vi "UHR-Fleezers Control (host) - 10.7.vi"() -> ()   [LabVIEW 2011] (continued)
        n1255 = Decrement(x="Scan steps (MCL)") -> (x-1=w1891:u64)
        n1256 = Divide(x="Scan Range (V)\n(of steps)", y=w1891) -> (x/y=w1890:dbl)
        "Desired Scan Incr (V)" <- w1890
        n1257 = local read "APD Integration Time (s)"() -> (w1883:dbl)
        n1258 = Multiply(x=w1890, y=w1870) -> (x*y=w1899:dbl)
        n1259 = Divide(x=w1899, y=10.0) -> (x/y=w1889:dbl)
        "Desired incr (int)" <- w1889
        n1260 = local read "Update Count (MCL)"() -> (w1895:u32)
        n1261 = Round Toward -Infinity(1:w1889) -> (0:w1898:dbl)
        n1262 = To Word Integer(number=w1898) -> (16bit integer=w1873:i16)
        "Actual Incr. int (MCL)" <- w1873
        n1263 = Multiply(x=w1883, y=40000000.0) -> (x*y=w1896:dbl)
        n1264 = Divide(x=w1896, y=w1895) -> (x/y=w1894:dbl)
        n1265 = Multiply(x=i16 10, y=w1873) -> (x*y=w1871:i16)
        n1266 = Multiply(x="N APD Samp/step", y=w1894) -> (x*y=w1893:dbl)
        "Cycles/step (MCL)" <- w1893
        n1267 = Divide(x=w1871, y=w1870) -> (x/y=→"Actual MCL Inc (V)":dbl)
        n1268 = Multiply(x="N APD Samp/step", y="Scan steps (MCL)") -> (x*y=w1885:dbl)
        n1269 = local read "APD Samples/FIFO Acq."() -> (w1882:dbl)
        n1270 = Multiply(x=w1885, y=u64 2) -> (x*y=w1884:dbl)
        "Data points/scan (f+b)" <- w1884
        n1271 = Multiply(x=w1884, y=w1875) -> (x*y=w1902:dbl)
        "Data points/scans (MCL)" <- w1902
        n1272 = Multiply(x=w1883, y=w1884) -> (x*y=w1876:dbl)
        "Time/f+b scan (s) (MCL)" <- w1876
        n1273 = Divide(x=w1902, y=w1882) -> (x/y=→"N sets should be saved (MCL)":dbl)
        n1274 = Multiply(x=w1876, y=w1875) -> (x*y=→"Total Time (s)":dbl)
        n1275 = Not(x="Fast Scan Dir") -> (.not. x?=w1880:bool)
        n1276 = xnode "Read/Write Control"("FPGA VI Reference In"=w1906, "error in"=w1905, "Scan steps (MCL)"="Scan steps (MCL)", "Number of scans (MCL)"=w1875, "Cycles per step (MCL)"=w1893, "Scan freq.  increment (MCL)"=w1873, "1D or 2D Scan?"="2D or 1D Scan", "MCL Scan Axis"=w1880, "Cont. Scan (MCL)"="Continuous MCL Scanning") -> ("error out"=w1904:errorcluster)  [unwired: 1 out]
      }
      event "Read Cal": Value Change {
        w1908 = 1000.0 ("y")
        n1277 = event-data() -> ()  [unwired: 7 out]
        n1278 = local read "Save file name"() -> (w1933:path)
        n1279 = local write "Read Cal"(FALSE ("Read Cal")) -> ()
        n1280 = Strip Path(path=w1933) -> (stripped path=w1932:path)  [unwired: 1 out]
        n1281 = Path To String(path=w1932) -> (string=w1931:string)
        n1282 = Concatenate Strings(w1931, "\\current.cal" ("string")) -> (w1929:string)
        n1283 = String To Path(string=w1929) -> (path=w1928:path)
        n1284 = Open/Create/Replace File(file path (use dialog)=w1928, operation (0:open)=T25."open", access (0:read/write)=enum16{"read/write", "read-only", "write-only"}."read-only") -> (refnum out=w1936:refnum<file>, error out=w1922:errorcluster)  [unwired: 1 in, 3 out]
        n1285 = Deny Access(4:w1922, 7:w1936) -> (0:w1921:errorcluster, 3:w1927:refnum<file>)  [unwired: 1 out]
        n1286 = Read from Binary File(5:0.0, 8:w1921, 9:T24."big-endian, network order" ("byte order (0:big-endian, network order)"), 10:-1 ("count (1)"), 11:w1927) -> (0:w1920:errorcluster, 2:w1918:dbl[], 3:w1923:refnum<file>)  [unwired: 2 out]
        n1287 = Array To Cluster(array=w1918) -> (cluster=w1917:T27)
        n1288 = Unbundle(w1917) -> ("[0]"=w1916:dbl, "[1]"=w1915:dbl, "[2]"=w1914:dbl, "[3]"=w1913:dbl, "[4]"=w1912:dbl, "[5]"=w1911:dbl)
        n1289 = Close File(refnum=w1923, error in=w1920) -> (error out=→"Read cal error":errorcluster)  [unwired: 1 out]
        n1290 = Multiply(x=w1911, y=w1908) -> (x*y=w1909:dbl)
        n1291 = local write "T2 kappa_x (pN/nm)"(w1913) -> ()
        n1292 = local write "T1 kappa_x (pN/nm)"(w1914) -> ()
        n1293 = local write "T1 alpha_x (nm/V)"(w1916) -> ()
        n1294 = local write "T2 alpha_x (nm/V)"(w1915) -> ()
        n1295 = Multiply(x=w1912, y=w1908) -> (x*y=w1910:dbl)
        n1296 = local write "T1 offset_x (mV)"(w1910) -> ()
        n1297 = local write "T2 offset_x (mV)"(w1909) -> ()
      }
      event "Abort MCL Scan": Value Change {
        n1298 = event-data() -> ()  [unwired: 7 out]
        n1299 = local write "MCL Scanning"(FALSE ("MCL Scanning")) -> ()
        n1300 = xnode "Read/Write Control"("FPGA VI Reference In"=w1941, "error in"=w1940, "Abort scan (MCL)"="Abort MCL Scan") -> ("error out"=w1939:errorcluster)  [unwired: 1 out]
      }
      event "Update Count (MCL)": Value Change {
        n1301 = event-data() -> ()  [unwired: 7 out]
        n1302 = xnode "Read/Write Control"("FPGA VI Reference In"=w1945, "error in"=w1944, "MCL count"="Update Count (MCL)") -> ("error out"=w1943:errorcluster)  [unwired: 1 out]
      }
      event "Phase adjust (MCL)", "+ phase (MCL)", "- phase (MCL)": Value Change {
        n1303 = event-data() -> ()  [unwired: 7 out]
        n1304 = Negate(x="Phase adjust (MCL)") -> (-x=w1954:i16)
        n1305 = Select(t=w1954, s="- phase (MCL)", f="Phase adjust (MCL)") -> (s? t:f=w1952:i16)
        n1306 = Or(x="- phase (MCL)", y="+ phase (MCL)") -> (x .or. y?=w1947:bool)
        n1307 = xnode "Read/Write Control"("FPGA VI Reference In"=w1956, "error in"=w1955, "Phase count adjustment (MCL)"=w1952) -> ("FPGA VI Reference Out"=w1948:T19, "error out"=w1949:errorcluster)
        n1308 = xnode "Read/Write Control"("FPGA VI Reference In"=w1948, "error in"=w1949, "+ phase (MCL)"=w1947) -> ("error out"=w1946:errorcluster)  [unwired: 1 out]
      }
      event "Abort AOD Scan": Value Change {
        n1309 = event-data() -> ()  [unwired: 7 out]
        n1310 = xnode "Read/Write Control"("FPGA VI Reference In"=w1960, "error in"=w1959, "Abort scan"="Abort AOD Scan") -> ("error out"=w1958:errorcluster)  [unwired: 1 out]
      }
      event "Continuous AOD Scanning": Value Change {
        n1311 = event-data() -> ()  [unwired: 7 out]
        n1312 = xnode "Read/Write Control"("FPGA VI Reference In"=w1964, "error in"=w1963, "Cont. Scan"="Continuous AOD Scanning") -> ("error out"=w1962:errorcluster)  [unwired: 1 out]
      }
      event "Index": Value Change {
        n1313 = event-data() -> ()  [unwired: 7 out]
        n1314 = call "Create new save file.vi"("Insert"="", "Ext"=".dat" ("string"), "Index In"="Index") -> ("Path Out"=→"Save file name":path, "Index Out"=w1965:dbl)
        "Save index" <- w1965
        n1315 = local write "Index"(w1965) -> ()
      }
      event "AO1", "AO2": Value Change {
        w1980 = 10.0 ("y")
        w1979 = 32767.0 ("y")
        n1316 = event-data() -> ()  [unwired: 7 out]
        n1317 = local read "AO2"() -> (w1978:dbl)
        n1318 = local read "AO1"() -> (w1975:dbl)
        n1319 = Multiply(x=w1975, y=w1979) -> (x*y=w1974:dbl)
        n1320 = Multiply(x=w1978, y=w1979) -> (x*y=w1977:dbl)
        n1321 = Divide(x=w1974, y=w1980) -> (x/y=w1973:dbl)
        n1322 = Divide(x=w1977, y=w1980) -> (x/y=w1976:dbl)
        n1323 = To Word Integer(number=w1973) -> (16bit integer=w1981:i16)
        n1324 = To Word Integer(number=w1976) -> (16bit integer=w1982:i16)
        n1325 = xnode "Read/Write Control"("FPGA VI Reference In"=w1972, "error in"=w1971, "AO1"=w1981, "AO2"=w1982) -> ("error out"=w1970:errorcluster)  [unwired: 1 out]
      }
      event "Inject Pump 1": Value Change {
        n1326 = event-data() -> ()  [unwired: 7 out]
        n1327 = local read "Use Harvard pumps\nfor beads (else Chemyx)"() -> (w1984:bool)
        n1328 = case shown="True" w1984 {
          tunnel: "Inject Pump 1" -> [w1988 w2026]
          tunnel: w1983 -> [_ w2027]
          frame False {
            n1329 = local read "Pump write delay (ms)"() -> (w1987:dbl)
            n1330 = local read "Chemyx Syringe Pump Serial Port"() -> (w1986:refnum<visa-resource-name>)
            n1331 = case shown="True" w1988 {
              tunnel: w1987 -> [w1994 w2008]
              tunnel: w1986 -> [w1991 w2007]
              frame False {
                n1332 = flat-sequence {
                  tunnel: w1991 -> [w1995]
                  tunnel: [w1995] -> w1992
                  tunnel: w1994 -> [_]
                  tunnel: [w1998] -> w1993
                  tunnel: w1992 -> [w1998]
                  tunnel: w1993 -> [w1999]
                  tunnel: [w1999] -> w1989
                  tunnel: [w2001] -> w1990
                  tunnel: w1989 -> [w2001]
                  tunnel: w1990 -> [w2003]
                  frame #0 {
                    n1333 = call "Write to pump.vi"("string"="enter pump1", "VISA resource name"=w1995) -> ()  [unwired: 1 out]
                  }
                  frame #1 {
                    n1334 = Wait (ms)(milliseconds to wait="Pump pause delay (ms)") -> ()  [unwired: 1 out]
                  }
                  frame #2 {
                    n1335 = call "Write to pump.vi"("string"="stop", "VISA resource name"=w1999) -> ()  [unwired: 1 out]
                  }
                  frame #3 {
                    n1336 = Wait (ms)(milliseconds to wait=u32 500) -> ()  [unwired: 1 out]
                  }
                  frame #4 {
                    n1337 = call "Write to pump.vi"("string"="stop", "VISA resource name"=w2003) -> ()  [unwired: 1 out]
                  }
                }
              }
              frame True {
                n1338 = flat-sequence {
                  tunnel: w2007 -> [w2017]
                  tunnel: w2008 -> [w2012]
                  tunnel: w2008 -> [w2019]
                  tunnel: w2007 -> [w2020]
                  tunnel: [w2020] -> w2005
                  tunnel: [w2022] -> w2006
                  tunnel: w2005 -> [w2022]
                  tunnel: w2006 -> [w2024]
                  frame #0 {
                    n1339 = local read "All Pump Parameters"() -> (w2011:T5)
                    n1340 = Unbundle By Name(w2011) -> ("Pump 1"=w2018:T28)
                    n1341 = call "Set pump parameters.vi"("Pump write delay (ms)"=w2012, "Volume (uL)"="Ch 1 Inject Volume (uL)", "Rate (uL/h)"="Ch 1 Inject Rate (ul/h)", "Units"=4.0, "Pump #"=1.0, "Pump Parameters In"=w2018, "VISA resource name"=w2017) -> ("Pump Parameters Out"=w2010:T28)  [unwired: 3 in]
                    n1342 = Bundle By Name(cluster=w2011, "Pump 1"=w2010) -> (w2009:T5)
                    n1343 = local write "All Pump Parameters"(w2009) -> ()
                  }
                  frame #1 {
                    n1344 = Wait (ms)(milliseconds to wait=w2019) -> ()  [unwired: 1 out]
                  }
                  frame #2 {
                    n1345 = call "Write to pump.vi"("string"="start", "VISA resource name"=w2020) -> ()  [unwired: 1 out]
                  }
                  frame #3 {
                    n1346 = Wait (ms)(milliseconds to wait=u32 500) -> ()  [unwired: 1 out]
                  }
                  frame #4 {
                    n1347 = call "Write to pump.vi"("string"="start", "VISA resource name"=w2024) -> ()  [unwired: 1 out]
                  }
                }
              }
            }
          }
          frame True {
            n1348 = case shown="False" w2026 {
              tunnel: w2027 -> [w2028 w2038]
              frame False {
                n1349 = flat-sequence {
                  tunnel: w2028 -> [w2030]
                  frame #0 {
                    n1350 = local write "Flushing P1"(FALSE ("Flushing P1")) -> ()
                    n1351 = Concatenate Strings("stop" ("string"), "\r") -> (w2032:string)
                    n1352 = VISA Write(VISA resource name=w2030, write buffer=w2032) -> ()  [unwired: 1 in, 3 out]
                  }
                  frame #1 {
                    n1353 = property on="Clear Volume P1" class="Bool (strict)"("Val(Sgnl)"=TRUE ("Value (Signaling)")) -> ()  [unwired: 2 in, 2 out]
                  }
                }
              }
              frame True {
                n1354 = local read "Normal Flow Rate (ul/h) P1"() -> (w2036:dbl)
                n1355 = Number To Decimal String(number=w2036) -> (decimal integer string=w2042:string)  [unwired: 1 in]
                n1356 = Concatenate Strings("irate  " ("string"), w2042, " u/h" ("string"), "\r") -> (w2040:string)
                n1357 = VISA Write(VISA resource name=w2038, write buffer=w2040) -> (VISA resource name out=w2037:refnum<visa-resource-name>)  [unwired: 1 in, 2 out]
                n1358 = Concatenate Strings("irun" ("string"), "\r") -> (w2044:string)
                n1359 = VISA Write(VISA resource name=w2037, write buffer=w2044) -> ()  [unwired: 1 in, 3 out]
              }
            }
          }
        }
      }
      event "Inject Pump 3": Value Change {
        n1360 = event-data() -> ()  [unwired: 7 out]
        n1361 = local read "Use Harvard pumps\nfor beads (else Chemyx)"() -> (w2047:bool)
        n1362 = case shown="True" w2047 {
          tunnel: "Inject Pump 3" -> [w2051 w2090]
          tunnel: w2046 -> [_ w2089]
          frame False {
            n1363 = local read "Pump write delay (ms)"() -> (w2050:dbl)
            n1364 = case shown="True" w2051 {
              tunnel: w2050 -> [w2057 w2071]
              tunnel: "Chemyx Syringe Pump Serial Port" -> [w2054 w2070]
              frame False {
                n1365 = flat-sequence {
                  tunnel: w2054 -> [w2058]
                  tunnel: [w2058] -> w2055
                  tunnel: w2057 -> [_]
                  tunnel: [w2061] -> w2056
                  tunnel: w2055 -> [w2061]
                  tunnel: w2056 -> [w2062]
                  tunnel: [w2062] -> w2052
                  tunnel: [w2064] -> w2053
                  tunnel: w2052 -> [w2064]
                  tunnel: w2053 -> [w2066]
                  frame #0 {
                    n1366 = call "Write to pump.vi"("string"="enter pump3", "VISA resource name"=w2058) -> ()  [unwired: 1 out]
                  }
                  frame #1 {
                    n1367 = local read "Pump pause delay (ms)"() -> (w2060:u32)
                    n1368 = Wait (ms)(milliseconds to wait=w2060) -> ()  [unwired: 1 out]
                  }
                  frame #2 {
                    n1369 = call "Write to pump.vi"("string"="stop", "VISA resource name"=w2062) -> ()  [unwired: 1 out]
                  }
                  frame #3 {
                    n1370 = Wait (ms)(milliseconds to wait=u32 0) -> ()  [unwired: 1 out]
                  }
                  frame #4 {
                    n1371 = call "Write to pump.vi"("string"="stop", "VISA resource name"=w2066) -> ()  [unwired: 1 out]
                  }
                }
              }
              frame True {
                n1372 = flat-sequence {
                  tunnel: w2070 -> [w2080]
                  tunnel: w2071 -> [w2075]
                  tunnel: w2071 -> [w2082]
                  tunnel: w2070 -> [w2083]
                  tunnel: [w2083] -> w2069
                  tunnel: [w2086] -> w2068
                  tunnel: w2069 -> [w2086]
                  tunnel: w2068 -> [w2087]
                  frame #0 {
                    n1373 = local read "All Pump Parameters"() -> (w2074:T5)
                    n1374 = Unbundle By Name(w2074) -> ("Pump 3"=w2081:T28)
                    n1375 = call "Set pump parameters.vi"("Pump write delay (ms)"=w2075, "Volume (uL)"="Ch 3 Inject Volume (uL)", "Rate (uL/h)"="Ch 3 Inject Rate (ul/h)", "Units"=4.0, "Pump #"=3.0, "Pump Parameters In"=w2081, "VISA resource name"=w2080) -> ("Pump Parameters Out"=w2073:T28)  [unwired: 3 in]
                    n1376 = Bundle By Name(cluster=w2074, "Pump 3"=w2073) -> (w2072:T5)
                    n1377 = local write "All Pump Parameters"(w2072) -> ()
                  }
                  frame #1 {
                    n1378 = Wait (ms)(milliseconds to wait=w2082) -> ()  [unwired: 1 out]
                  }
                  frame #2 {
                    n1379 = call "Write to pump.vi"("string"="start", "VISA resource name"=w2083) -> ()  [unwired: 1 out]
                  }
                  frame #3 {
                    n1380 = Wait (ms)(milliseconds to wait=u32 500) -> ()  [unwired: 1 out]
                  }
                  frame #4 {
                    n1381 = call "Write to pump.vi"("string"="start", "VISA resource name"=w2087) -> ()  [unwired: 1 out]
                  }
                }
              }
            }
          }
          frame True {
            n1382 = case shown="False" w2090 {
              tunnel: w2089 -> [w2091 w2098]
              frame False {
                n1383 = flat-sequence {
                  tunnel: w2091 -> [w2093]
                  frame #0 {
                    n1384 = local write "Flushing P3"(FALSE ("Flushing P3")) -> ()
                    n1385 = Concatenate Strings("stop" ("string"), "\r") -> (w2095:string)
                    n1386 = VISA Write(VISA resource name=w2093, write buffer=w2095) -> ()  [unwired: 1 in, 3 out]
                  }
                  frame #1 {
                    n1387 = property on="Clear Volume P3" class="Bool (strict)"("Val(Sgnl)"=TRUE ("Value (Signaling)")) -> ()  [unwired: 2 in, 2 out]
                  }
                }
              }
              frame True {
                n1388 = local read "Normal Flow Rate (ul/h) P3"() -> (w2099:dbl)
                n1389 = Number To Decimal String(number=w2099) -> (decimal integer string=w2105:string)  [unwired: 1 in]
                n1390 = Concatenate Strings("irate  " ("string"), w2105, " u/h" ("string"), "\r") -> (w2103:string)
                n1391 = VISA Write(VISA resource name=w2098, write buffer=w2103) -> (VISA resource name out=w2101:refnum<visa-resource-name>)  [unwired: 1 in, 2 out]
                n1392 = Concatenate Strings("irun" ("string"), "\r") -> (w2107:string)
                n1393 = VISA Write(VISA resource name=w2101, write buffer=w2107) -> ()  [unwired: 1 in, 3 out]
              }
            }
          }
        }
      }
      event "Inject Pump 2": Value Change {
        n1394 = event-data() -> ()  [unwired: 7 out]
        n1395 = local read "Pump write delay (ms)"() -> (w2111:dbl)
        n1396 = flat-sequence {
          tunnel: w2109 -> [w2124]
          tunnel: w2111 -> [w2120]
          tunnel: "Inject Pump 2" -> [_]
          tunnel: w2111 -> [w2126]
          tunnel: w2109 -> [w2127]
          frame #0 {
            n1397 = local read "All Pump Parameters"() -> (w2119:T5)
            n1398 = Multiply(x=60.0, y="Flush Center Ch Rate (ul/m)") -> (x*y=w2116:dbl)
            n1399 = Unbundle By Name(w2119) -> ("Pump 2"=w2125:T28)
            n1400 = call "Set pump parameters.vi"("Pump write delay (ms)"=w2120, "Volume (uL)"="Flush Center Ch Volume (uL)", "Rate (uL/h)"=w2116, "Units"=3.0, "Pump #"=2.0, "Pump Parameters In"=w2125, "VISA resource name"=w2124) -> ("Pump Parameters Out"=w2118:T28)  [unwired: 3 in]
            n1401 = Bundle By Name(cluster=w2119, "Pump 2"=w2118) -> (w2117:T5)
            n1402 = local write "All Pump Parameters"(w2117) -> ()
            n1403 = Add(x="Flush Center Ch Volume (uL)", y="Total Volume\nFlushed (uL)") -> (x+y=w2113:dbl)
            n1404 = local write "Total Volume\nFlushed (uL)"(w2113) -> ()
          }
          frame #1 {
            n1405 = Wait (ms)(milliseconds to wait=w2126) -> ()  [unwired: 1 out]
          }
          frame #2 {
            n1406 = call "Write to pump.vi"("string"="start", "VISA resource name"=w2127) -> ()  [unwired: 1 out]
          }
        }
        n1407 = local read "Chemyx Syringe Pump Serial Port"() -> (w2109:refnum<visa-resource-name>)
      }
      event "Sample Channel\nFlow": Value Change {
        n1408 = event-data() -> ()  [unwired: 7 out]
        n1409 = Select(t="irun" ("string"), s="Sample Channel\nFlow", f="stop" ("string")) -> (s? t:f=w2131:string)
        n1410 = Concatenate Strings(w2131, "\r") -> (w2134:string)
        n1411 = VISA Write(VISA resource name=w2129, write buffer=w2134) -> ()  [unwired: 1 in, 3 out]
      }
      event "Start Flow": Value Change {
        n1412 = event-data() -> ()  [unwired: 7 out]
        n1413 = local write "Sample Channel\nFlow"(TRUE ("Sample Channel\nFlow")) -> ()
        n1414 = local write "Start Flow"(FALSE ("Start Flow")) -> ()
        n1415 = Concatenate Strings("irun" ("string"), "\r") -> (w2140:string)
        n1416 = VISA Write(VISA resource name=w2136, write buffer=w2140) -> ()  [unwired: 1 in, 3 out]
      }
      event "Stop Flow": Value Change {
        w2142 = FALSE ("Stop Flow")
        n1417 = event-data() -> ()  [unwired: 7 out]
        n1418 = local write "Stop Flow"(w2142) -> ()
        n1419 = local write "Sample Channel\nFlow"(w2142) -> ()
        n1420 = Concatenate Strings("stop" ("string"), "\r") -> (w2145:string)
        n1421 = VISA Write(VISA resource name=w2143, write buffer=w2145) -> ()  [unwired: 1 in, 3 out]
      }
      event "Flow rate (uL/h)": Value Change {
        n1422 = event-data() -> ()  [unwired: 7 out]
        n1423 = Number To Decimal String(number="Flow rate (uL/h)") -> (decimal integer string=w2152:string)  [unwired: 1 in]
        n1424 = Concatenate Strings("irate  " ("string"), w2152, " u/h" ("string"), "\r") -> (w2151:string)
        n1425 = VISA Write(VISA resource name=w2148, write buffer=w2151) -> ()  [unwired: 1 in, 3 out]
      }
      event "Flush Sample": Value Change {
        n1426 = event-data() -> ()  [unwired: 7 out]
        n1427 = flat-sequence {
          tunnel: w2157 -> [w2185]
          tunnel: [w2165] -> w2156
          tunnel: [w2159] -> w2154
          tunnel: w2156 -> [w2189]
          tunnel: [w2189] -> w2155
          tunnel: w2154 -> [w2188]
          tunnel: w2155 -> [w2194]
          frame #0 {
            # "set paramaters (rate, volume) for flush, clear volume"
            n1428 = Number To Decimal String(number="Flush rate (uL/m)") -> (decimal integer string=w2181:string)  [unwired: 1 in]
            n1429 = Concatenate Strings("irate  " ("string"), w2181, " u/m" ("string"), "\r") -> (w2183:string)
            n1430 = VISA Write(VISA resource name=w2185, write buffer=w2183) -> (VISA resource name out=w2179:refnum<visa-resource-name>)  [unwired: 1 in, 2 out]
            n1431 = Reciprocal(x="Flush rate (uL/m)") -> (1/x=w2162:dbl)
            n1432 = Number To Decimal String(number="Volume (uL)") -> (decimal integer string=w2170:string)  [unwired: 1 in]
            n1433 = Multiply(x="Volume (uL)", y=w2162) -> (x*y=w2161:dbl)
            n1434 = Concatenate Strings("tvolume  " ("string"), w2170, " u" ("string"), "\r") -> (w2168:string)
            n1435 = Multiply(x=w2161, y=60000.0) -> (x*y=w2159:dbl)
            n1436 = VISA Write(VISA resource name=w2179, write buffer=w2168) -> (VISA resource name out=w2167:refnum<visa-resource-name>)  [unwired: 1 in, 2 out]
            n1437 = Concatenate Strings("cvolume" ("string"), "\r") -> (w2166:string)
            n1438 = VISA Write(VISA resource name=w2167, write buffer=w2166) -> (VISA resource name out=w2177:refnum<visa-resource-name>)  [unwired: 1 in, 2 out]
            n1439 = Concatenate Strings("irun" ("string"), "\r") -> (w2175:string)
            n1440 = VISA Write(VISA resource name=w2177, write buffer=w2175) -> (VISA resource name out=w2165:refnum<visa-resource-name>)  [unwired: 1 in, 2 out]
          }
          frame #1 {
            # "Have to wait until\nflow is done to reset\nrate"
            n1441 = Add(x=w2188, y=100.0) -> (x+y=w2187:dbl)
            n1442 = Wait (ms)(milliseconds to wait=w2187) -> ()  [unwired: 1 out]
          }
          frame #2 {
            # "reset flow rate to usual flow rate"
            n1443 = local read "Flow rate (uL/h)"() -> (w2200:dbl)
            n1444 = Number To Decimal String(number=w2200) -> (decimal integer string=w2198:string)  [unwired: 1 in]
            n1445 = Concatenate Strings("irate  " ("string"), w2198, " u/h" ("string"), "\r") -> (w2196:string)
            n1446 = VISA Write(VISA resource name=w2194, write buffer=w2196) -> (VISA resource name out=w2190:refnum<visa-resource-name>)  [unwired: 1 in, 2 out]
            n1447 = Concatenate Strings("cvolume" ("string"), "\r") -> (w2191:string)
            n1448 = VISA Write(VISA resource name=w2190, write buffer=w2191) -> ()  [unwired: 1 in, 3 out]
          }
        }
      }
      event "Flush Pump 3": Value Change {
        n1449 = event-data() -> ()  [unwired: 7 out]
        n1450 = flat-sequence {
          tunnel: w2201 -> [w2204]
          frame #0 {
            # "set paramaters (rate, volume) for flush, clear volume"
            n1451 = Number To Decimal String(number="Flush rate (uL/m) P3") -> (decimal integer string=w2226:string)  [unwired: 1 in]
            n1452 = local write "Inject Pump 3"(TRUE ("Inject Pump 3")) -> ()
            n1453 = Concatenate Strings("irate  " ("string"), w2226, " u/m" ("string"), "\r") -> (w2228:string)
            n1454 = VISA Write(VISA resource name=w2204, write buffer=w2228) -> (VISA resource name out=w2224:refnum<visa-resource-name>)  [unwired: 1 in, 2 out]
            n1455 = Reciprocal(x="Flush rate (uL/m) P3") -> (1/x=w2208:dbl)
            n1456 = Number To Decimal String(number="Volume (uL) P3") -> (decimal integer string=w2215:string)  [unwired: 1 in]
            n1457 = Multiply(x="Volume (uL) P3", y=w2208) -> (x*y=w2207:dbl)
            n1458 = Concatenate Strings("tvolume  " ("string"), w2215, " u" ("string"), "\r") -> (w2213:string)
            n1459 = Multiply(x=w2207, y=60.0) -> (x*y=→"HP3 Flush Time (s)":dbl)
            n1460 = VISA Write(VISA resource name=w2224, write buffer=w2213) -> (VISA resource name out=w2212:refnum<visa-resource-name>)  [unwired: 1 in, 2 out]
            n1461 = Concatenate Strings("cvolume" ("string"), "\r") -> (w2211:string)
            n1462 = VISA Write(VISA resource name=w2212, write buffer=w2211) -> (VISA resource name out=w2222:refnum<visa-resource-name>)  [unwired: 1 in, 2 out]
            n1463 = Concatenate Strings("irun" ("string"), "\r") -> (w2220:string)
            n1464 = VISA Write(VISA resource name=w2222, write buffer=w2220) -> ()  [unwired: 1 in, 3 out]
          }
          frame #1 {
            "Flushing P3" <- TRUE ("Flushing P3")
          }
        }
      }
      event "Flush Pump 1": Value Change {
        n1465 = event-data() -> ()  [unwired: 7 out]
        n1466 = flat-sequence {
          tunnel: [w2242] -> w2232
          tunnel: w2231 -> [w2235]
          tunnel: w2232 -> [_]
          frame #0 {
            # "set paramaters (rate, volume) for flush, clear volume"
            n1467 = local write "Inject Pump 1"(TRUE ("Inject Pump 1")) -> ()
            n1468 = Number To Decimal String(number="Flush rate (uL/m) P1") -> (decimal integer string=w2258:string)  [unwired: 1 in]
            n1469 = Concatenate Strings("irate  " ("string"), w2258, " u/m" ("string"), "\r") -> (w2260:string)
            n1470 = VISA Write(VISA resource name=w2235, write buffer=w2260) -> (VISA resource name out=w2256:refnum<visa-resource-name>)  [unwired: 1 in, 2 out]
            n1471 = Reciprocal(x="Flush rate (uL/m) P1") -> (1/x=w2239:dbl)
            n1472 = Number To Decimal String(number="Volume (uL) P1") -> (decimal integer string=w2247:string)  [unwired: 1 in]
            n1473 = Multiply(x="Volume (uL) P1", y=w2239) -> (x*y=w2238:dbl)
            n1474 = Concatenate Strings("tvolume  " ("string"), w2247, " u" ("string"), "\r") -> (w2245:string)
            n1475 = Multiply(x=w2238, y=60.0) -> (x*y=→"HP1 Flush Time (s)":dbl)
            n1476 = VISA Write(VISA resource name=w2256, write buffer=w2245) -> (VISA resource name out=w2244:refnum<visa-resource-name>)  [unwired: 1 in, 2 out]
            n1477 = Concatenate Strings("cvolume" ("string"), "\r") -> (w2243:string)
            n1478 = VISA Write(VISA resource name=w2244, write buffer=w2243) -> (VISA resource name out=w2254:refnum<visa-resource-name>)  [unwired: 1 in, 2 out]
            n1479 = Concatenate Strings("irun" ("string"), "\r") -> (w2252:string)
            n1480 = VISA Write(VISA resource name=w2254, write buffer=w2252) -> (VISA resource name out=w2242:refnum<visa-resource-name>)  [unwired: 1 in, 2 out]
          }
          frame #1 {
            "Flushing P1" <- TRUE ("Flushing P3")
          }
        }
      }
      event "Clear Volume": Value Change {
        n1481 = event-data() -> ()  [unwired: 7 out]
        n1482 = Concatenate Strings("cvolume" ("string"), "\r") -> (w2264:string)
        n1483 = VISA Write(VISA resource name=w2263, write buffer=w2264) -> ()  [unwired: 1 in, 3 out]
      }
      event "Clear Volume P3": Value Change {
        n1484 = event-data() -> ()  [unwired: 7 out]
        n1485 = Concatenate Strings("cvolume" ("string"), "\r") -> (w2270:string)
        n1486 = VISA Write(VISA resource name=w2269, write buffer=w2270) -> ()  [unwired: 1 in, 3 out]
        n1487 = local write "Clear Volume P3"(FALSE ("Clear Volume P3")) -> ()
      }
      event "Clear Volume P1": Value Change {
        n1488 = event-data() -> ()  [unwired: 7 out]
        n1489 = Concatenate Strings("cvolume" ("string"), "\r") -> (w2275:string)
        n1490 = local write "Clear Volume P1"(FALSE ("Clear Volume P1")) -> ()
        n1491 = VISA Write(VISA resource name=w2274, write buffer=w2275) -> ()  [unwired: 1 in, 3 out]
      }
      event "Display On P3": Value Change {
        n1492 = event-data() -> ()  [unwired: 7 out]
        n1493 = Select(t="dim 100", s="Display On P3", f="dim 0") -> (s? t:f=w2281:string)
        n1494 = Concatenate Strings(w2281, "\r") -> (w2283:string)
        n1495 = VISA Write(VISA resource name=w2278, write buffer=w2283) -> ()  [unwired: 1 in, 3 out]
      }
      event "Display On P1": Value Change {
        n1496 = event-data() -> ()  [unwired: 7 out]
        n1497 = Select(t="dim 100", s="Display On P1", f="dim 0") -> (s? t:f=w2288:string)
        n1498 = Concatenate Strings(w2288, "\r") -> (w2290:string)
        n1499 = VISA Write(VISA resource name=w2285, write buffer=w2290) -> ()  [unwired: 1 in, 3 out]
      }
      event "Retract Pump 3": Value Change {
        n1500 = event-data() -> ()  [unwired: 7 out]
        n1501 = local write "Retract Pump 3"(FALSE ("Retract Pump 3")) -> ()
        n1502 = case shown="True" "Retract Pump 3" {
          tunnel: w2292 -> [_ w2295]
          frame False {
          }
          frame True {
            n1503 = Number To Decimal String(number="Retract Rate (uL/m)") -> (decimal integer string=w2313:string)  [unwired: 1 in]
            n1504 = Concatenate Strings("wrate  " ("string"), w2313, " u/m" ("string"), "\r") -> (w2315:string)
            n1505 = VISA Write(VISA resource name=w2295, write buffer=w2315) -> (VISA resource name out=w2306:refnum<visa-resource-name>)  [unwired: 1 in, 2 out]
            n1506 = Number To Decimal String(number="Retract Vol 3 (uL)") -> (decimal integer string=w2308:string)  [unwired: 1 in]
            n1507 = Concatenate Strings("tvolume  " ("string"), w2308, " u" ("string"), "\r") -> (w2305:string)
            n1508 = VISA Write(VISA resource name=w2306, write buffer=w2305) -> (VISA resource name out=w2301:refnum<visa-resource-name>)  [unwired: 1 in, 2 out]
            n1509 = Concatenate Strings("cvolume" ("string"), "\r") -> (w2302:string)
            n1510 = VISA Write(VISA resource name=w2301, write buffer=w2302) -> (VISA resource name out=w2296:refnum<visa-resource-name>)  [unwired: 1 in, 2 out]
            n1511 = Concatenate Strings("wrun" ("string"), "\r") -> (w2297:string)
            n1512 = VISA Write(VISA resource name=w2296, write buffer=w2297) -> ()  [unwired: 1 in, 3 out]
          }
        }
      }
      event "Retract Pump 1": Value Change {
        n1513 = event-data() -> ()  [unwired: 7 out]
        n1514 = local write "Retract Pump 1"(FALSE ("Retract Pump 1")) -> ()
        n1515 = case shown="True" "Retract Pump 1" {
          tunnel: w2317 -> [_ w2322]
          frame False {
          }
          frame True {
            n1516 = local read "Retract Rate (uL/m)"() -> (w2320:dbl)
            n1517 = Number To Decimal String(number=w2320) -> (decimal integer string=w2338:string)  [unwired: 1 in]
            n1518 = Concatenate Strings("wrate  " ("string"), w2338, " u/m" ("string"), "\r") -> (w2340:string)
            n1519 = VISA Write(VISA resource name=w2322, write buffer=w2340) -> (VISA resource name out=w2332:refnum<visa-resource-name>)  [unwired: 1 in, 2 out]
            n1520 = Number To Decimal String(number="Retract Vol 1 (uL)") -> (decimal integer string=w2334:string)  [unwired: 1 in]
            n1521 = Concatenate Strings("tvolume  " ("string"), w2334, " u" ("string"), "\r") -> (w2331:string)
            n1522 = VISA Write(VISA resource name=w2332, write buffer=w2331) -> (VISA resource name out=w2328:refnum<visa-resource-name>)  [unwired: 1 in, 2 out]
            n1523 = Concatenate Strings("cvolume" ("string"), "\r") -> (w2329:string)
            n1524 = VISA Write(VISA resource name=w2328, write buffer=w2329) -> (VISA resource name out=w2323:refnum<visa-resource-name>)  [unwired: 1 in, 2 out]
            n1525 = Concatenate Strings("wrun" ("string"), "\r") -> (w2324:string)
            n1526 = VISA Write(VISA resource name=w2323, write buffer=w2324) -> ()  [unwired: 1 in, 3 out]
          }
        }
      }
      event "Flip Green Filter": Value Change {
        n1527 = event-data() -> ()  [unwired: 7 out]
        n1528 = Not(x="Flip Green Filter") -> (.not. x?=w2342:bool)
        n1529 = local write "Flip Green Filter"(w2342) -> ()
        n1530 = flat-sequence {
          tunnel: w2350 -> [w2355]
          tunnel: w2349 -> [w2354]
          tunnel: [w2352] -> w2347
          tunnel: [w2351] -> w2346
          tunnel: [w2357] -> w2345
          tunnel: w2347 -> [w2357]
          tunnel: [w2356] -> w2344
          tunnel: w2346 -> [w2356]
          tunnel: w2345 -> [w2361]
          tunnel: w2344 -> [w2360]
          tunnel: [w2359] -> w2348
          frame #0 {
            n1531 = xnode "Read/Write Control"("FPGA VI Reference In"=w2355, "error in"=w2354, "Green Filter Flipper"=TRUE) -> ("FPGA VI Reference Out"=w2352:T19, "error out"=w2351:errorcluster)
          }
          frame #1 {
            n1532 = Wait (ms)(milliseconds to wait=u32 100) -> ()  [unwired: 1 out]
          }
          frame #2 {
            n1533 = xnode "Read/Write Control"("FPGA VI Reference In"=w2361, "error in"=w2360, "Green Filter Flipper"=FALSE) -> ("error out"=w2359:errorcluster)  [unwired: 1 out]
          }
        }
      }
      event "Pump 1 contents", "Pump 3 contents": Value Change {
        n1534 = event-data() -> ()  [unwired: 7 out]
        n1535 = local read "Pump 1 contents"() -> (→"Pump 1 cont disp":string)
        n1536 = local read "Pump 3 contents"() -> (→"Pump 3 cont disp":string)
      }
      event "Reset Trap Pos. FB": Value Change {
        n1537 = event-data() -> ()  [unwired: 7 out]
        n1538 = xnode "Read/Write Control"("FPGA VI Reference In"=w2367, "error in"=w2366, "Trap Pos. FB Reset"="Reset Trap Pos. FB") -> ()  [unwired: 2 out]
      }
      event "Rem fb disp offset": Value Change {
        n1539 = event-data() -> ()  [unwired: 7 out]
        n1540 = local write "Rem fb disp offset"(FALSE ("Rem fb disp offset")) -> ()
        n1541 = local read "Mean T1 Position (nm)"() -> (w2369:dbl)
        n1542 = local read "FB Trap Pos Offset"() -> (w2370:dbl)
        n1543 = Subtract(x=w2370, y=w2369) -> (x-y=w2368:dbl)
        n1544 = local write "FB Trap Pos Offset"(w2368) -> ()
      }
      event "Threshold (nm)": Value Change {
        n1545 = event-data() -> ()  [unwired: 7 out]
        n1546 = flat-sequence {
          tunnel: w2374 -> [w2382]
          tunnel: w2373 -> [w2381]
          tunnel: [w2375] -> w2372
          tunnel: w2372 -> [w2388]
          frame #0 {
            n1547 = xnode "Read/Write Control"("FPGA VI Reference In"=w2382, "error in"=w2381) -> ("FPGA VI Reference Out"=w2378:T19, "error out"=w2377:errorcluster, "FPGA TTrig Thresh"=w2379:i64)
            n1548 = local read "Threshold stored (nm)"() -> (w2387:dbl)
            n1549 = local read "Threshold (nm)"() -> (w2375:dbl)
            n1550 = local read "AOM X Cal (nm/MHz)"() -> (w2385:dbl)
            n1551 = Subtract(x=w2375, y=w2387) -> (x-y=w2386:dbl)
            n1552 = Divide(x=w2386, y=w2385) -> (x/y=w2383:dbl)
            n1553 = call "IR AOM freq to word.vi"("Frequency In (MHz)"=w2383) -> ("Frequency Word Out (double)"=w2384:dbl)
            n1554 = To Quad Integer(1:w2384) -> (0:w2380:i64)
            n1555 = Add(x=w2379, y=w2380) -> (x+y=w2376:i64)
            n1556 = xnode "Read/Write Control"("FPGA VI Reference In"=w2378, "error in"=w2377, "FPGA TTrig Thresh"=w2376) -> ()  [unwired: 2 out]
          }
          frame #1 {
            "Threshold stored (nm)" <- w2388
          }
        }
      }
      event "FB Trig Integrate": Value Change {
        n1557 = event-data() -> ()  [unwired: 7 out]
        n1558 = local read "FB Trig Integrate"() -> (w2390:u32)
        n1559 = xnode "Read/Write Control"("FPGA VI Reference In"=w2392, "error in"=w2391, "FB Trig Integrate"=w2390) -> ("error out"=w2389:errorcluster)  [unwired: 1 out]
      }
      event "11": Value Change {
        n1560 = event-data() -> ()  [unwired: 7 out]
        n1561 = local read "11"() -> (w2393:bool)
        n1562 = case shown="True" w2393 {
          frame False {
          }
          frame True {
            n1563 = local read "Messages"() -> (w2395:string)
            n1564 = call "Update messages.vi"("Message to add"="You kicked it up to 11!", "Old message string"=w2395) -> ("New message string"=w2396:string)
            n1565 = call <vilib>:"Beep.vi"() -> ()  [unwired: 12 in]
            n1566 = local write "Messages"(w2396) -> ()
          }
        }
      }
      event "Trap Pos. FB ON": Value Change {
        n1567 = event-data() -> ()  [unwired: 7 out]
        n1568 = xnode "Read/Write Control"("FPGA VI Reference In"=w2399, "error in"=w2398, "Force feedback"="Trap Pos. FB ON") -> ()  [unwired: 2 out]
      }
      event "Remove Action Offset": Value Change {
        n1569 = event-data() -> ()  [unwired: 7 out]
        n1570 = local write "Remove Action Offset"(FALSE ("Remove Action Offset")) -> ()
        n1571 = local read "Trap Pos. FB Mult Factor"() -> (w2404:i64)
        n1572 = local read "Trap Pos FB Action"() -> (w2402:i64)
        n1573 = local read "Trap Pos. FB Offset Factor"() -> (w2400:i64)
        n1574 = Multiply(x=w2404, y=w2402) -> (x*y=w2403:i64)
        n1575 = Add(x=w2403, y=w2400) -> (x+y=w2401:i64)
        n1576 = local write "Trap Pos. FB Offset Factor"(w2401) -> ()
        n1577 = xnode "Read/Write Control"("FPGA VI Reference In"=w2407, "error in"=w2406, "Trap Pos. FB Offset Factor"=w2401) -> ()  [unwired: 2 out]
      }
      event "Remove Unwinding Offset": Value Change {
        n1578 = event-data() -> ()  [unwired: 7 out]
        n1579 = local write "Remove Unwinding Offset"(FALSE ("Remove Action Offset")) -> ()
        n1580 = local read "Trap Pos. FB Mult Factor"() -> (w2419:i64)
        n1581 = local read "Trap Pos FB Action"() -> (w2417:i64)
        n1582 = local read "Trap Pos. FB Offset Factor"() -> (w2416:i64)
        n1583 = Multiply(x=w2419, y=w2417) -> (x*y=w2418:i64)
        n1584 = local read "Trap Pos. FB Mult Factor"() -> (w2415:i64)
        n1585 = Add(x=w2418, y=w2416) -> (x+y=w2409:i64)
        n1586 = Multiply(x=32768, y="factor") -> (x*y=w2412:dbl)
        n1587 = Multiply(x=w2412, y=w2415) -> (x*y=w2414:dbl)
        n1588 = Subtract(x=w2409, y=w2414) -> (x-y=w2413:dbl)
        n1589 = To Quad Integer(1:w2413) -> (0:w2408:i64)
        n1590 = xnode "Read/Write Control"("FPGA VI Reference In"=w2422, "error in"=w2421, "Trap Pos. FB Offset Factor"=w2408) -> ()  [unwired: 2 out]
        n1591 = local write "Trap Pos. FB Offset Factor"(w2408) -> ()
      }
      event "Trap Pos. FB Range", "Trap Pos. FB Gains", "Trap Pos. FB Mult Factor", "Trap Pos. FB Offset Factor", "Trap Pos FB Negate Action", "Trap Pos FB Monitor\nT1 or T2", "Differential FB?", "Negate Diff?": Value Change {
        n1592 = event-data() -> ()  [unwired: 7 out]
        n1593 = local read "Negate Diff?"() -> (w2423:bool)
        n1594 = xnode "Read/Write Control"("FPGA VI Reference In"=w2433, "error in"=w2432, "Trap Pos. FB Range"="Trap Pos. FB Range", "Trap Pos. FB Gains"="Trap Pos. FB Gains", "Trap Pos. FB Mult Factor"="Trap Pos. FB Mult Factor", "Trap Pos. FB Offset Factor"="Trap Pos. FB Offset Factor", "Trap Pos FB Negate Action"="Trap Pos FB Negate Action", "Trap Pos FB Monitor T1 or T2"="Trap Pos FB Monitor\nT1 or T2", "AI1 X Scale"="Trap Pos. AI1 X Pre-scale", "Negate Diff?"=w2423, "Diff FB Measurement?"="Differential FB?") -> ()  [unwired: 2 out]
      }
      event "Trap Pos FB SP": Value Change {
        n1595 = event-data() -> ()  [unwired: 7 out]
        n1596 = xnode "Read/Write Control"("FPGA VI Reference In"=w2436, "error in"=w2435, "Trap Pos. FB SP"="Trap Pos FB SP") -> ()  [unwired: 2 out]
      }
      event "Set Reading to\nSetpoint": Value Change {
        # "This is the actual PID input signal"
        n1597 = event-data() -> ()  [unwired: 7 out]
        n1598 = local write "Set Reading to\nSetpoint"(FALSE ("Set SP to Reading")) -> ()
        n1599 = xnode "Read/Write Control"("FPGA VI Reference In"=w2441, "error in"=w2440) -> ("FPGA VI Reference Out"=w2439:T19, "error out"=w2438:errorcluster, "Trap Pos FB Int-Norm Signal"=w2437:fxp<+/-,16,1>)
        n1600 = local read "Differential FB?"() -> (w2442:bool)
        n1601 = case shown="False" w2442 {
          tunnel: [w2447 w2454] -> w2444
          tunnel: w2437 -> [w2445 w2454]
          frame False {
            n1602 = local read "Trap Pos FB Monitor\nT1 or T2"() -> (w2450:bool)
            n1603 = local read "Trap X AI1 (DMA)"() -> (w2453:T13)
            n1604 = Unbundle By Name(w2453) -> ("Set 1"=w2452:fxp<+/-,16,1>, "Set 2"=w2451:fxp<+/-,16,1>)
            n1605 = Select(t=w2452, s=w2450, f=w2451) -> (s? t:f=w2449:fxp<+/-,16,1>)
            n1606 = Not(x="Set SP Using...") -> (.not. x?=w2446:bool)
            n1607 = Select(t=w2445, s=w2446, f=w2449) -> (s? t:f=w2447:fxp<+/-,16,1>)
          }
          frame True {
          }
        }
        n1608 = xnode "Read/Write Control"("FPGA VI Reference In"=w2439, "error in"=w2438, "Trap Pos. FB SP"=w2444) -> ()  [unwired: 2 out]
        n1609 = local write "Trap Pos FB SP"(w2444) -> ()
      }
      event "Trap Pos. FB Out Scale 2^n": Value Change {
        n1610 = event-data() -> ()  [unwired: 7 out]
        n1611 = Scale By Power Of 2(n="Trap Pos. FB Out Scale 2^n", x=ext 1.0) -> (x*2^n=w2455:ext)
        n1612 = property on="Trap Pos. FB Mult Factor" class="DigNum (strict)"("Val(Sgnl)"=w2455) -> ()  [unwired: 2 in, 2 out]
      }
      event "Trap Pos FB Int Count": Value Change {
        n1613 = event-data() -> ()  [unwired: 7 out]
        n1614 = xnode "Read/Write Control"("FPGA VI Reference In"=w2460, "error in"=w2459, "Trap Pos FB Int Count"="Trap Pos FB Int Count") -> ()  [unwired: 2 out]
      }
    }
    "error out 2" <- w1373
    n1615 = node-c288() -> ()  [unwired: 2 out]
  }
  n1616 = timed-loop "Mouse control: trap position (AOM deflection), set confocal spot from image" {
    tunnel: [w2462] -> w182
    tunnel: w50 -> [w2461]
    timing: w94 -> [_]
    timing-out: [_] -> w93
    stop <- w2462 stop-if-true
    n1617 = node-c288() -> ()  [unwired: 2 out]
    n1618 = event shown="[0] \"Pane\": Mouse Down" {
      selector: _ -> [_ _]
      dyn-events: _ -> [_ _]
      timeout: _ -> [_ _]
      tunnel: w2461 -> [w2465 _]
      event Mouse Down {
        n1619 = event-data() -> ("Time"=w2467:u32, "Coords"=w2466:T7, "Button"=w2468:u16)  [unwired: 6 out]
        n1620 = case shown="1" w2468 {
          tunnel: w2467 -> [_ _ w2571]
          tunnel: w2466 -> [_ w2505 w2569]
          tunnel: w2465 -> [_ _ w2567]
          frame 0, Default {
          }
          frame 1 {
            n1621 = property on="APD 2" class="ImageControl"() -> ("Displayed Image Position"=w2475:cluster{"Left":i32, "Top":i32})  [unwired: 2 in, 2 out]
            n1622 = property on="APD 1" class="ImageControl"() -> ("Displayed Image Position"=w2504:cluster{"Left":i32, "Top":i32})  [unwired: 2 in, 2 out]
            n1623 = property on="Detection Laser X" class="ImageControl"() -> ("Displayed Image Position"=w2501:cluster{"Left":i32, "Top":i32})  [unwired: 2 in, 2 out]
            n1624 = property on="Detection Laser Y" class="ImageControl"() -> ("Displayed Image Position"=w2500:cluster{"Left":i32, "Top":i32})  [unwired: 2 in, 2 out]
            n1625 = property on="APD 2" class="ImageControl"() -> ("Displayed Image Size"=w2474:cluster{"Width":u32, "Height":u32})  [unwired: 2 in, 2 out]
            n1626 = property on="APD 1" class="ImageControl"() -> ("Displayed Image Size"=w2502:cluster{"Width":u32, "Height":u32})  [unwired: 2 in, 2 out]
            n1627 = property on="Detection Laser X" class="ImageControl"() -> ("Displayed Image Size"=w2503:cluster{"Width":u32, "Height":u32})  [unwired: 2 in, 2 out]
            n1628 = property on="Detection Laser Y" class="ImageControl"() -> ("Displayed Image Size"=w2499:cluster{"Width":u32, "Height":u32})  [unwired: 2 in, 2 out]
            n1629 = Unbundle By Name(w2474) -> ("Width"=w2471:u32, "Height"=w2470:u32)
            n1630 = Unbundle By Name(w2475) -> ("Left"=w2473:i32, "Top"=w2472:i32)
            n1631 = Unbundle By Name(w2502) -> ("Width"=w2496:u32, "Height"=w2495:u32)
            n1632 = Unbundle By Name(w2503) -> ("Width"=w2492:u32, "Height"=w2491:u32)
            n1633 = Unbundle By Name(w2499) -> ("Width"=w2488:u32, "Height"=w2487:u32)
            n1634 = Unbundle By Name(w2504) -> ("Left"=w2498:i32, "Top"=w2497:i32)
            n1635 = Unbundle By Name(w2501) -> ("Left"=w2494:i32, "Top"=w2493:i32)
            n1636 = Unbundle By Name(w2500) -> ("Left"=w2490:i32, "Top"=w2489:i32)
            n1637 = Bundle("Left"=w2473, "Top"=w2472, "Width"=w2471, "Height"=w2470) -> (w2469:T29)  [unwired: 1 in]
            n1638 = Bundle("Left"=w2498, "Top"=w2497, "Width"=w2496, "Height"=w2495) -> (w2486:T29)  [unwired: 1 in]
            n1639 = Bundle("Left"=w2494, "Top"=w2493, "Width"=w2492, "Height"=w2491) -> (w2485:T29)  [unwired: 1 in]
            n1640 = Bundle("Left"=w2490, "Top"=w2489, "Width"=w2488, "Height"=w2487) -> (w2484:T29)  [unwired: 1 in]
            n1641 = Build Cluster Array(w2469, w2486, w2485, w2484) -> (w2483:T30)
            n1642 = for {
              tunnel: w2505 -> [w2516]
              tunnel: w2483 -> [w2517] mode=indexing
              shift-right: [w2514] -> w2481
              shift-left: TRUE -> [w2515]
              shift-right: [w2513] -> w2479
              shift-left: _ -> [w2509]
              shift-right: [w2512] -> w2478
              shift-left: _ -> [w2508]
              shift-right: [w2511] -> w2477
              shift-left: _ -> [w2507]
              shift-right: [w2510] -> w2476
              shift-left: _ -> [w2506]
              n1643 = case shown="True" w2515 {
                selector: w2515 -> [w2522 _]
                tunnel: w2517 -> [_ w2531]
                tunnel: w2516 -> [_ w2529]
                tunnel: [w2522 w2527] -> w2514
                tunnel: [w2521 w2526] -> w2513
                tunnel: [w2520 w2525] -> w2512
                tunnel: [w2519 w2524] -> w2511
                tunnel: [w2518 w2523] -> w2510
                tunnel: w2509 -> [w2521 _]
                tunnel: w2508 -> [w2520 _]
                tunnel: w2507 -> [w2519 _]
                tunnel: w2506 -> [w2518 _]
                frame False {
                }
                frame True {
                  n1644 = Unbundle(w2531) -> (w2530:T29)
                  n1645 = call "isclickinwindow.vi"("Image Param"=w2530, "Point32"=w2529) -> ("4 Y"=w2523:i32, "3 Height"=w2524:i32, "2 X"=w2525:i32, "1 Width"=w2526:i32, "In image?"=w2528:bool)  [unwired: 1 in]
                  n1646 = Not(x=w2528) -> (.not. x?=w2527:bool)
                }
              }
            }
            n1647 = Not(x=w2481) -> (.not. x?=w2480:bool)
            n1648 = case shown="True" w2480 {
              tunnel: w2478 -> [_ w2544]
              tunnel: w2476 -> [_ w2543]
              tunnel: w2479 -> [_ w2542]
              tunnel: w2477 -> [_ w2541]
              frame False {
              }
              frame True {
                w2537 = FALSE ("Get Point")
                n1649 = local read "Scan lines (y)"() -> (w2546:u64)
                n1650 = local read "Actual MCL Inc (V)"() -> (w2538:dbl)
                n1651 = local read "Scan steps (MCL)"() -> (w2545:u64)
                n1652 = Divide "Y Pix/step"(x=w2541, y=w2546) -> (x/y=w2553:dbl)
                n1653 = Divide "Y V/pix"(x=w2538, y=w2553) -> (x/y=w2552:dbl)
                n1654 = Divide "Y half step offset"(x=w2538, y=2.0) -> (x/y=w2554:dbl)
                n1655 = Divide "X pix/step"(x=w2542, y=w2545) -> (x/y=w2551:dbl)
                n1656 = Negate(x=w2554) -> (-x=w2555:dbl)
                n1657 = local read "Initial Y"() -> (w2561:dbl)
                n1658 = Multiply(x=w2543, y=w2552) -> (x*y=w2562:dbl)
                n1659 = Divide "X half step offset"(x=w2538, y=2.0) -> (x/y=w2548:dbl)
                n1660 = Divide "X V/pix"(x=w2538, y=w2551) -> (x/y=w2550:dbl)
                n1661 = Multiply(x=w2538, y=w2545) -> (x*y=w2557:dbl)
                n1662 = Compound Arithmetic op=ADD(w2555, w2562, w2561) -> (w2539:dbl)
                "Pointer Y (V)" <- w2539
                n1663 = Multiply(x=w2550, y=w2544) -> (x*y=w2559:dbl)
                n1664 = Negate(x=w2548) -> (-x=w2547:dbl)
                n1665 = local read "Initial X"() -> (w2560:dbl)
                n1666 = Negate(x=w2559) -> (-x=w2558:dbl)
                n1667 = Compound Arithmetic op=ADD(w2547, w2557, w2560, w2558) -> (w2540:dbl)
                "Pointer X (V)" <- w2540
                n1668 = Or(x="Set X Only", y="Set Confocal Spot (X-Y)") -> (x .or. y?=w2533:bool)
                n1669 = Or(x="Set Confocal Spot (X-Y)", y="Set Y Only") -> (x .or. y?=w2532:bool)
                n1670 = case shown="True" w2533 {
                  tunnel: w2540 -> [_ w2563]
                  frame False {
                  }
                  frame True {
                    n1671 = property on="AO2" class="Slide (strict)"("Val(Sgnl)"=w2563) -> ()  [unwired: 2 in, 2 out]
                  }
                }
                n1672 = case shown="True" w2532 {
                  tunnel: w2539 -> [_ w2564]
                  frame False {
                  }
                  frame True {
                    n1673 = property on="AO1" class="Slide (strict)"("Val(Sgnl)"=w2564) -> ()  [unwired: 2 in, 2 out]
                  }
                }
                n1674 = local write "Set Confocal Spot (X-Y)"(w2537) -> ()
                n1675 = local write "Set X Only"(w2537) -> ()
                n1676 = local write "Set Y Only"(w2537) -> ()
              }
            }
          }
          frame 3 {
            n1677 = local read "BD 2 Frequency 1 (MHz)"() -> (w2565:dbl)
            n1678 = local read "BD 1 Frequency 1 (MHz)"() -> (w2566:dbl)
            n1679 = local write "Manipulating Trap"(TRUE ("Manipulating Trap")) -> ()
            n1680 = local write "Coords"(T7 {"Horizontal"=0, "Vertical"=0} ("Coords")) -> ()
            n1681 = while {
              tunnel: w2571 -> [w2576]
              tunnel: w2569 -> [w2575]
              tunnel: w2567 -> [w2574]
              tunnel: w2566 -> [w2573]
              tunnel: w2565 -> [w2572]
              stop <- w2577 stop-if-true
              n1682 = event shown="[0] \"Pane\": Mouse Move" {
                selector: _ -> [_ _]
                dyn-events: _ -> [_ _]
                timeout: _ -> [_ _]
                tunnel: ["Force Manip Abort" w2641] -> w2577
                tunnel: w2576 -> [w2584 _]
                tunnel: w2575 -> [w2582 _]
                tunnel: w2574 -> [w2581 _]
                tunnel: w2573 -> [w2580 _]
                tunnel: w2572 -> [w2579 _]
                event Mouse Move {
                  n1683 = event-data() -> ("Time"=w2585:u32, "Coords"=w2586:T7)  [unwired: 3 out]
                  n1684 = Less?(x=w2585, y=w2584) -> (x < y?=w2583:bool)
                  n1685 = case "Makes sure old motion events prior to mouse click aren't used" shown="False" w2583 {
                    tunnel: w2586 -> [w2628 _]
                    tunnel: w2582 -> [w2629 _]
                    tunnel: w2581 -> [w2606 _]
                    tunnel: w2580 -> [w2602 _]
                    tunnel: w2579 -> [w2601 _]
                    frame False {
                      n1686 = Subtract(x=w2628, y=w2629) -> (x-y=w2627:T7)
                      "Coords" <- w2627
                      n1687 = local read "Y RF Frequency Limits (MHz)"() -> (w2587:T16)
                      n1688 = To Double Precision Float(number=w2627) -> (double precision float=w2626:cluster{"Horizontal":dbl, "Vertical":dbl})
                      n1689 = Multiply(x=cluster{"Horizontal":dbl, "Vertical":dbl} {"Horizontal"=-1.0, "Vertical"=1.0}, y="Manipulation Scaling") -> (x*y=w2622:cluster{"Horizontal":dbl, "Vertical":dbl})
                      n1690 = local read "X RF Frequency Limits (MHz)"() -> (w2588:T16)
                      n1691 = Multiply(x=w2626, y=w2622) -> (x*y=w2624:cluster{"Horizontal":dbl, "Vertical":dbl})
                      n1692 = Unbundle By Name(w2624) -> ("Horizontal"=w2619:dbl, "Vertical"=w2623:dbl)
                      n1693 = Unbundle By Name(w2587) -> ("Maximum"=w2590:dbl, "Minimum"=w2589:dbl)
                      n1694 = Boolean To (0,1)(Boolean="Manip. X?") -> (0, 1=w2617:i16)
                      n1695 = Boolean To (0,1)(Boolean="Manip. Y?") -> (0, 1=w2614:i16)
                      n1696 = local read "BD 1 Frequency 2 (MHz)"() -> (w2604:dbl)
                      n1697 = Multiply(x=w2623, y=w2614) -> (x*y=w2616:dbl)
                      n1698 = Multiply(x=w2617, y=w2619) -> (x*y=w2620:dbl)
                      n1699 = local read "BD 2 Frequency 2 (MHz)"() -> (w2603:dbl)
                      n1700 = Unbundle By Name(w2588) -> ("Maximum"=w2592:dbl, "Minimum"=w2591:dbl)
                      n1701 = Add(x=w2601, y=w2616) -> (x+y=w2594:dbl)
                      n1702 = Add(x=w2602, y=w2620) -> (x+y=w2596:dbl)
                      n1703 = In Range and Coerce(upper limit=w2592, x=w2596, lower limit=w2591) -> (coerced(x)=w2595:dbl)  [unwired: 1 out]
                      n1704 = In Range and Coerce(upper limit=w2590, x=w2594, lower limit=w2589) -> (coerced(x)=w2593:dbl)  [unwired: 1 out]
                      n1705 = Subtract(x=w2595, y=w2604) -> (x-y=w2613:dbl)
                      n1706 = Subtract(x=w2593, y=w2603) -> (x-y=w2612:dbl)
                      n1707 = Square(x=w2613) -> (x^2=w2611:dbl)
                      n1708 = Square(x=w2612) -> (x^2=w2610:dbl)
                      n1709 = Add(x=w2611, y=w2610) -> (x+y=w2609:dbl)
                      n1710 = Square Root(x=w2609) -> (sqrt(x)=w2605:dbl)
                      n1711 = In Range and Coerce(upper limit="Limit Max (MHz)", x=w2605, lower limit="Limit Min (MHz)") -> (In Range?=w2598:bool)  [unwired: 1 out]
                      n1712 = Not(x="Limits Enable") -> (.not. x?=w2597:bool)
                      n1713 = Or(x=w2598, y=w2597) -> (x .or. y?=w2599:bool)
                      n1714 = case shown="True" w2599 {
                        tunnel: w2606 -> [_ w2639]
                        tunnel: w2605 -> [_ w2630]
                        tunnel: w2595 -> [_ w2637]
                        tunnel: w2604 -> [_ w2636]
                        tunnel: w2593 -> [_ w2635]
                        tunnel: w2603 -> [_ w2634]
                        tunnel: w2588 -> [_ w2632]
                        tunnel: w2587 -> [_ w2631]
                        frame False {
                        }
                        frame True {
                          n1715 = local read "BD 1 Frequency 3 (MHz)"() -> (w2638:dbl)
                          n1716 = local read "BD 2 Frequency 3 (MHz)"() -> (w2633:dbl)
                          n1717 = local write "Trap Delta (MHz)"(w2630) -> ()
                          n1718 = call "set RF board frequency - interlace.vi"("Board 2 Frequency Limits"=w2631, "Board 1 Frequency Limits"=w2632, "FPGA VI Reference In"=w2639, "Board 2 Frequency 3 (MHz)"=w2633, "Board 1 Frequency 3 (MHz)"=w2638, "Board 2 Frequency 2 (MHz)"=w2634, "Board 2 Frequency 1 (MHz)"=w2635, "Board 1 Frequency 2 (MHz)"=w2636, "Board 1 Frequency 1  (MHz)"=w2637) -> ()  [unwired: 1 in, 2 out]
                          n1719 = local write "BD 2 Frequency 1 (MHz)"(w2635) -> ()
                          n1720 = local write "BD 1 Frequency 1 (MHz)"(w2637) -> ()
                        }
                      }
                    }
                    frame True {
                    }
                  }
                }
                event Mouse Up {
                  n1721 = event-data() -> ("Button"=w2640:u16)  [unwired: 8 out]
                  n1722 = case shown="3" w2640 {
                    tunnel: [FALSE TRUE] -> w2641
                    frame 0, Default {
                    }
                    frame 3 {
                      n1723 = local read "Trap Delta (MHz)"() -> (w2643:dbl)
                      n1724 = property on="Initial delta (MHz)" class="DigNum (strict)"("Val(Sgnl)"=w2643) -> ()  [unwired: 2 in, 2 out]
                      n1725 = local write "Manipulating Trap"(FALSE ("Manipulating Trap")) -> ()
                    }
                  }
                }
              }
            }
          }
        }
      }
      event Mouse Move {
        n1726 = event-data() -> ()  [unwired: 6 out]
      }
    }
    n1727 = local read "Stop All"() -> (w2462:bool)
    n1728 = node-c288() -> ()  [unwired: 2 out]
  }
  n1729 = flat-sequence "Video" {
    tunnel: [w2654] -> w80
    tunnel: w80 -> [w2695]
    frame #0 {
      n1730 = while {
        stop <- w2647 continue-if-true
        n1731 = call "Close Video Capture.vi"() -> ("error code OUT"=w2649:i32)
